vi "svfa_Wrap or Unwrap Phase (array).vi"(7 "phase units":T1, 9 "custom wrap range":T3={"minimum phase"=-180.0, "maximum phase"=180.0}, 10 "desired wrapping":T2(ring), 11 "phase in":dbl[](array[numeric])) -> (3 "phase out":dbl[](array[numeric]), 5 "unit label":string)   [LabVIEW 2017]
uses:
  <vilib>/addons/_NISVFA/_Shared subVIs/Controls/svc_Complimentary Spectrum Units.ctl
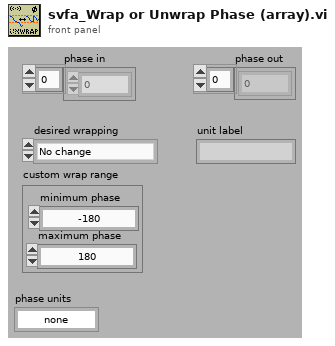
[diagram p1: front panel]
types:
  T1 = typedef "svc_Complimentary Spectrum Units.ctl" = enum16{"none", "radians", "degrees", "cycles", "imaginary"}
  T2 = enum16{"No change", "Unwrap", "Wrap: -360 to 0", "Wrap: -270 to 90", "Wrap: -180 to 180", "Wrap: -90 to 270", "Wrap: 0 to 360", "Wrap: custom range"}
  T3 = cluster{"minimum phase":dbl, "maximum phase":dbl}
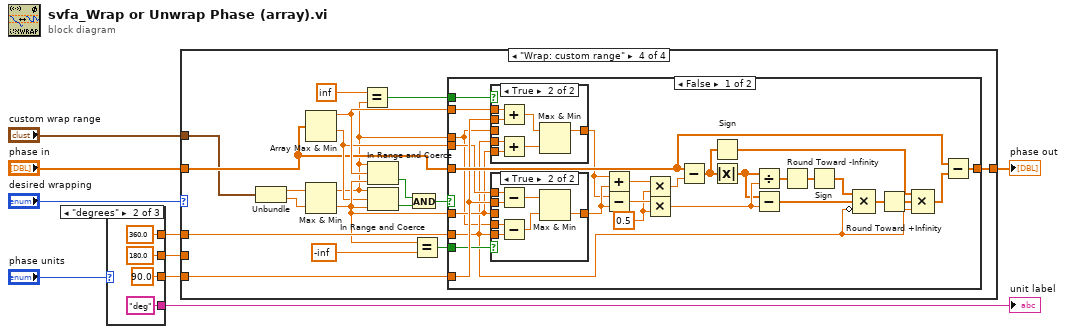
[diagram p0: block diagram]
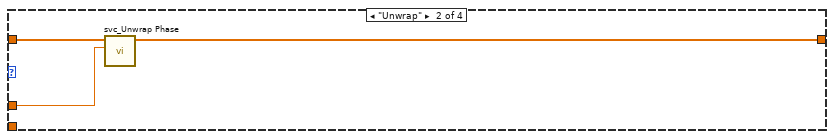
[diagram p3: hidden frame]
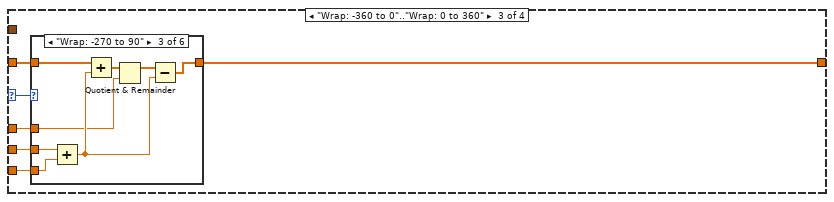
[diagram p4: hidden frame]
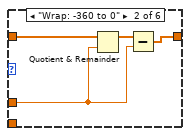
[diagram p6: hidden frame]
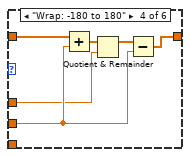
[diagram p7: hidden frame]
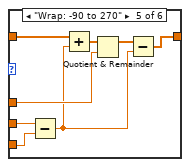
[diagram p8: hidden frame]
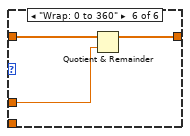
[diagram p9: hidden frame]
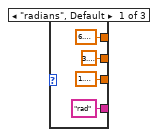
[diagram p13: hidden frame]
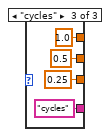
[diagram p14: hidden frame]
diagram:
  n1 = case shown="\"degrees\"" "phase units" {
    tunnel: [6.283185307179586 ("Pi Multiplied By 2") 360.0 1.0] -> w5
    tunnel: [3.141592653589793 ("Pi") 180.0 0.5] -> w4
    tunnel: [1.5707963267948966 ("Pi Divided By 2") 90.0 0.25] -> w6
    tunnel: ["rad" ("unit label") "deg" ("unit label") "cycles" ("unit label")] -> w7
    frame "radians", Default {
    }
    frame "degrees" {
    }
    frame "cycles" {
    }
  }
  "unit label" <- w7
  n2 = case shown="\"Wrap: custom range\"" "desired wrapping" {
    selector: "desired wrapping" -> [_ _ w29 _]
    tunnel: w4 -> [_ _ w30 _]
    tunnel: w5 -> [_ w25 w28 w74]
    tunnel: w6 -> [_ _ w31 w76]
    tunnel: "phase in" -> [w22 w24 w27 w64]
    tunnel: [w22 w23 w26 w77] -> w9
    tunnel: "custom wrap range" -> [_ _ _ w62]
    frame "No change", Default {
    }
    frame "Unwrap" {
      n3 = call <vilib>:"svc_Unwrap Phase.vi"("full cycle (2pi)"=w25, "phase in"=w24) -> ("phase out"=w23:dbl[])  [unwired: 8 in, 1 out]
    }
    frame "Wrap: -360 to 0".."Wrap: 0 to 360" {
      n4 = case shown="\"Wrap: -270 to 90\"" w29 {
        tunnel: w31 -> [_ _ w44 _ w57 _]
        tunnel: w30 -> [_ _ w39 w46 w58 _]
        tunnel: w27 -> [w32 w34 w41 w48 w54 w61]
        tunnel: [w32 w35 w40 w47 w53 w59] -> w26
        tunnel: w28 -> [_ w33 w37 w45 w52 w60]
        frame Default {
        }
        frame "Wrap: -360 to 0" {
          n5 = Quotient & Remainder(x=w34, y=w33) -> (x-y*floor(x/y)=w36:dbl[])  [unwired: 1 out]
          n6 = Subtract(x=w36, y=w33) -> (x-y=w35:dbl[])
        }
        frame "Wrap: -270 to 90" {
          n7 = Add(x=w39, y=w44) -> (x+y=w38:dbl)
          n8 = Add(x=w41, y=w38) -> (x+y=w42:dbl[])
          n9 = Quotient & Remainder(x=w42, y=w37) -> (x-y*floor(x/y)=w43:dbl[])  [unwired: 1 out]
          n10 = Subtract(x=w43, y=w38) -> (x-y=w40:dbl[])
        }
        frame "Wrap: -180 to 180" {
          n11 = Add(x=w48, y=w46) -> (x+y=w49:dbl[])
          n12 = Quotient & Remainder(x=w49, y=w45) -> (x-y*floor(x/y)=w50:dbl[])  [unwired: 1 out]
          n13 = Subtract(x=w50, y=w46) -> (x-y=w47:dbl[])
        }
        frame "Wrap: -90 to 270" {
          n14 = Subtract(x=w58, y=w57) -> (x-y=w51:dbl)
          n15 = Add(x=w54, y=w51) -> (x+y=w55:dbl[])
          n16 = Quotient & Remainder(x=w55, y=w52) -> (x-y*floor(x/y)=w56:dbl[])  [unwired: 1 out]
          n17 = Subtract(x=w56, y=w51) -> (x-y=w53:dbl[])
        }
        frame "Wrap: 0 to 360" {
          n18 = Quotient & Remainder(x=w61, y=w60) -> (x-y*floor(x/y)=w59:dbl[])  [unwired: 1 out]
        }
      }
    }
    frame "Wrap: custom range" {
      n19 = Unbundle(w62) -> ("minimum phase"=w79:dbl, "maximum phase"=w78:dbl)
      n20 = Array Max & Min(array=w64) -> (max value=w75:dbl, min value=w65:dbl)  [unwired: 2 out]
      n21 = Max & Min(x=w79, y=w78) -> (max(x,y)=w63:dbl, min(x,y)=w67:dbl)
      n22 = Equal?(x=inf, y=w63) -> (x = y?=w69:bool)
      n23 = In Range and Coerce(upper limit=w63, x=w75, lower limit=w67) -> (In Range?=w71:bool)  [unwired: 1 out]
      n24 = In Range and Coerce(upper limit=w63, x=w65, lower limit=w67) -> (In Range?=w72:bool)  [unwired: 1 out]
      n25 = And(x=w71, y=w72) -> (x .and. y?=w73:bool)
      n26 = Equal?(x=w67, y=-inf ("x")) -> (x = y?=w66:bool)
      n27 = case shown="False" w73 {
        tunnel: [w91 w123] -> w77
        tunnel: w64 -> [w90 w123]
        tunnel: w76 -> [w89 _]
        tunnel: w75 -> [w85 _]
        tunnel: w74 -> [w81 _]
        tunnel: w67 -> [w83 _]
        tunnel: w63 -> [w80 _]
        tunnel: w65 -> [w88 _]
        tunnel: w69 -> [w82 _]
        tunnel: w66 -> [w87 _]
        frame False {
          w103 = 0.5 ("y")
          n28 = case shown="True" w82 {
            tunnel: w89 -> [_ w114]
            tunnel: w85 -> [_ w113]
            tunnel: [w107 w111] -> w84
            tunnel: w83 -> [_ w109]
            tunnel: w81 -> [_ w108]
            tunnel: w80 -> [w107 _]
            frame False {
            }
            frame True {
              n29 = Add(x=w113, y=w114) -> (x+y=w110:dbl)
              n30 = Add(x=w108, y=w109) -> (x+y=w112:dbl)
              n31 = Max & Min(x=w110, y=w112) -> (max(x,y)=w111:dbl)  [unwired: 1 out]
            }
          }
          n32 = case shown="True" w87 {
            tunnel: w89 -> [_ w122]
            tunnel: w88 -> [_ w121]
            tunnel: [w115 w118] -> w86
            tunnel: w83 -> [w115 _]
            tunnel: w80 -> [_ w119]
            tunnel: w81 -> [_ w117]
            frame False {
            }
            frame True {
              n33 = Subtract(x=w121, y=w122) -> (x-y=w120:dbl)
              n34 = Subtract(x=w119, y=w117) -> (x-y=w116:dbl)
              n35 = Max & Min(x=w120, y=w116) -> (min(x,y)=w118:dbl)  [unwired: 1 out]
            }
          }
          n36 = Add(x=w84, y=w86) -> (x+y=w105:dbl)
          n37 = Subtract(x=w84, y=w86) -> (x-y=w106:dbl)
          n38 = Multiply(x=w105, y=w103) -> (x*y=w104:dbl)
          n39 = Multiply(x=w106, y=w103) -> (x*y=w102:dbl)
          n40 = Subtract(x=w90, y=w104) -> (x-y=w100:dbl[])
          n41 = Sign(1:w100) -> (0:w93:dbl[])
          n42 = Absolute Value(x=w100) -> (abs(x)=w92:dbl[])
          n43 = Divide(x=w92, y=w102) -> (x/y=w96:dbl[])
          n44 = Subtract(x=w92, y=w102) -> (x-y=w98:dbl[])
          n45 = Round Toward -Infinity ("Round To -Infinity")(1:w96) -> (0:w99:dbl[])
          n46 = Sign(1:w99) -> (0:w95:dbl[])
          n47 = Compound Arithmetic op=MULTIPLY(w95, w98, invert w81) -> (w94:dbl[])
          n48 = Round Toward +Infinity ("Round To +Infinity")(x=w94) -> (ceil(x): smallest int >= x=w97:dbl[])
          n49 = Compound Arithmetic op=MULTIPLY(w93, w97, w81) -> (w101:dbl[])
          n50 = Subtract(x=w90, y=w101) -> (x-y=w91:dbl[])
        }
        frame True {
        }
      }
    }
  }
  "phase out" <- w9
